vi "Triggered Broadcast.vi"(8 "error in":errorcluster, 9 "current time":timestamp, 10 "Triggered?":bool) -> (0 "error out":errorcluster)   [LabVIEW 2020, in "Sensor checking module.lvlib"]
doc: "Broadcast when simulated signal being True\n_____\nCreated using DQMH Event Scripter 7.0.1.1316."
uses:
  Sensor checking module.lvlib
  Triggered Broadcast Argument--cluster.ctl
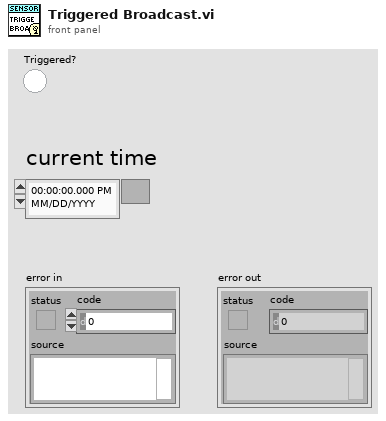
[diagram p1: front panel]
types:
  T1 = typedef "Sensor checking module.lvlib/Triggered Broadcast Argument--cluster.ctl" = cluster{"Triggered?":bool, "current time":timestamp}
  T2 = typedef "Sensor checking module.lvlib/Broadcast Events--cluster.ctl" = cluster{"Module Did Init":refnum<user-event>, "Status Updated":refnum<user-event>, "Error Reported":refnum<user-event>, "Module Did Stop":refnum<user-event>, "Update Module Execution Status":refnum<user-event>, "Triggered Broadcast":refnum<user-event>}
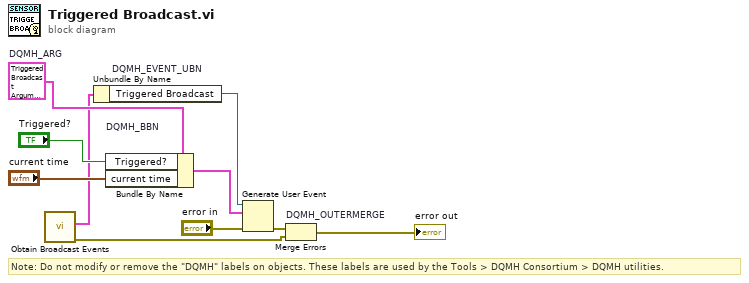
[diagram p0: block diagram]
diagram:
  w5 = T1 {"Triggered?"=FALSE, "current time"=timestamp(0 s since 1904-01-01)}  # DQMH_ARG
  # "Note: Do not modify or remove the \"DQMH\" labels on objects. These labels are used by the Tools > DQMH Consortium > DQMH utilities."
  n1 = call "Obtain Broadcast Events.vi"() -> ("error out"=w2:errorcluster, "Sensor checking module Broadcast Events"=w1:T2)  [unwired: 10 in]
  n2 = Unbundle By Name "DQMH_EVENT_UBN"(w1) -> ("Triggered Broadcast"=w7:refnum<user-event>)
  n3 = Bundle By Name "DQMH_BBN"(cluster=w5, "Triggered?"="Triggered?", "current time"="current time") -> (w8:T1)
  n4 = Generate User Event(user event=w7, event data cluster=w8, error in="error in") -> (error out=w6:errorcluster)  [unwired: 1 in, 1 out]
  n5 = Merge Errors "DQMH_OUTERMERGE"(w6, w2) -> (→"error out":errorcluster)
